vi "subReplaceAmpersandForXML.vi"(1 "String":string) -> (0 "result string":string)   [LabVIEW 2020, in "DefaultExtensions.lvlib" / "CGrapherDGML.lvclass"]
uses:
  CGrapherDGML.lvclass
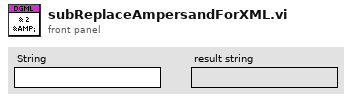
[diagram p1: front panel]
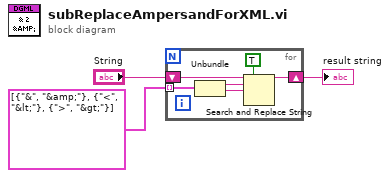
[diagram p0: block diagram]
diagram:
  n1 = for {
    shift-right: [w7] -> w2
    shift-left: "String" -> [w9]
    tunnel: cluster{string, string}[] [{"&", "&amp;"}, {"<", "&lt;"}, {">", "&gt;"}] -> [w6] mode=indexing
    n2 = Unbundle(w6) -> (w5:string, w4:string)
    n3 = Search and Replace String(replace all?=TRUE ("replace all? (F)"), input string=w9, search string=w5, replace string=w4) -> (result string=w7:string)  [unwired: 4 in, 3 out]
  }
  "result string" <- w2
